vi "UI_Main.vi"() -> ()   [LabVIEW 2014]
panel:
  out "Resultant Vector":T1
  out "SpeedCap":dbl(slide) scale=0.18..1.0
  out "Pod Data Out":T2(array[cluster])
  in  "Speed Constraints":T3
  out "FZ":dbl(slide) scale=-1.0..1.0
  out "FXY":cluster{"X":dbl, "Y":dbl}[](graph)
  out "Swerve":picture
  in  "Pod Coordinates":cluster{"X":dbl, "Y":dbl}[](array[cluster])=[{"X"=2.0, "Y"=2.0}, {"X"=2.0, "Y"=-2.0}, {"X"=-2.0, "Y"=2.0}, {"X"=-2.0, "Y"=-2.0}]
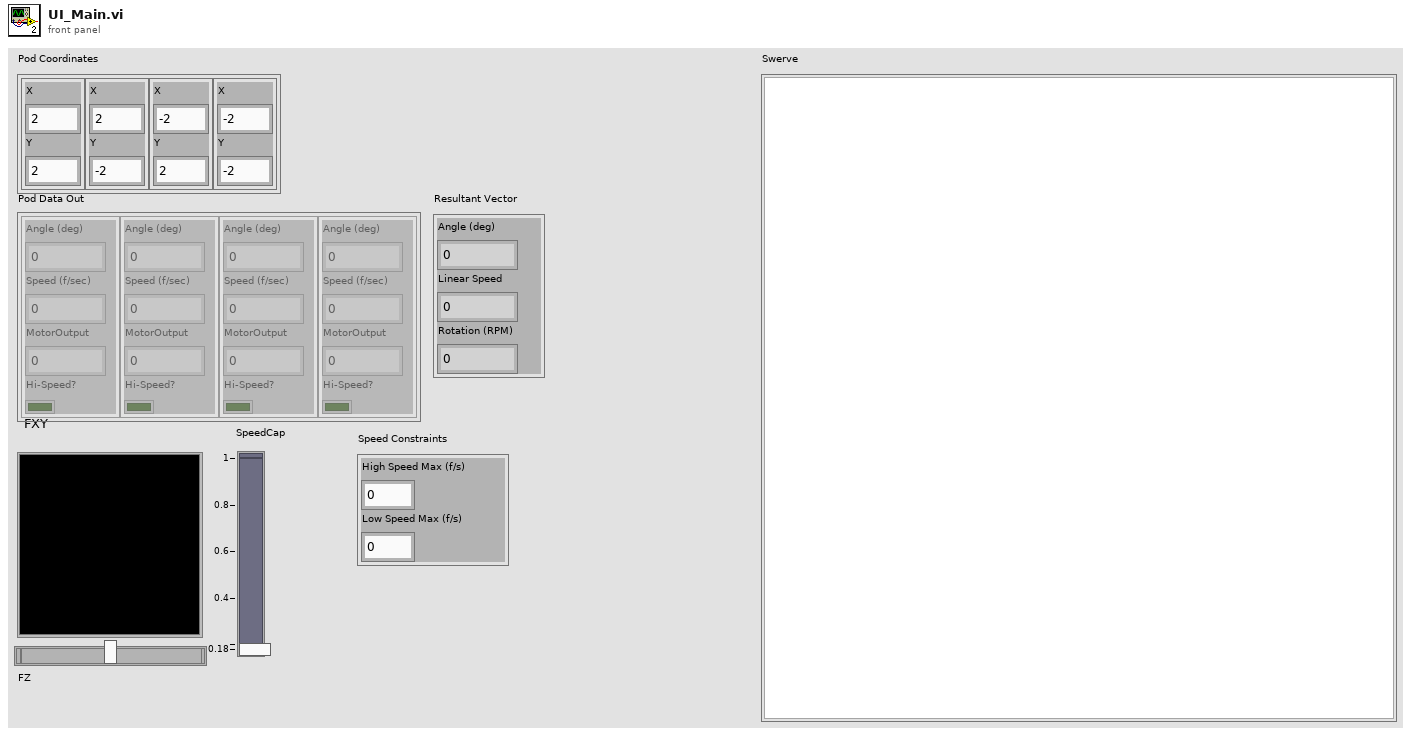
[diagram p1: front panel]
types:
  T1 = cluster{"Angle (deg)":dbl, "Linear Speed":dbl, "Rotation (RPM)":dbl}
  T2 = cluster{"Angle (deg)":dbl, "Speed (f/sec)":dbl, "MotorOutput":dbl, "Hi-Speed?":bool}[]
  T3 = cluster{"High Speed Max (f/s)":dbl, "Low Speed Max (f/s)":dbl}
  T4 = cluster{"Coords":cluster{"X":dbl, "Y":dbl}, "Vector":cluster{"X":dbl, "Y":dbl}, "Hi-Speed?":bool}[]
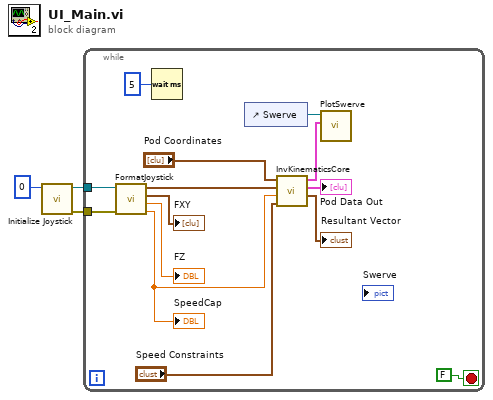
[diagram p0: block diagram]
diagram:
  n1 = call <vilib>:"Initialize Joystick.vi"("device index"=0) -> ("error out"=w1:errorcluster, "device ID"=w2:refnum<k1>)  [unwired: 9 in]
  n2 = while {
    tunnel: w2 -> [w14]
    tunnel: w1 -> [w13]
    stop <- FALSE stop-if-true
    n3 = call "FormatJoystick.vi"("error in (no error)"=w13, "Refnum in"=w14) -> ("Speed Cap"=w5:dbl, "FZ"=→"FZ":dbl, "FXY"=→"FXY":cluster{"X":dbl, "Y":dbl}[], "Axes"=w11:cluster{"X":dbl, "Y":dbl, "Z":dbl})  [unwired: 6 in]
    "SpeedCap" <- w5
    n4 = Wait (ms)(milliseconds to wait=u32 5) -> ()  [unwired: 1 out]
    n5 = control-ref of="Swerve"() -> (w17:refnum<vi>)
    n6 = call "InvKinematicsCore.vi"("Speed Constraints"="Speed Constraints", "Speed Cap"=w5, "Joystick Data"=w11, "Pod Coordinates"="Pod Coordinates") -> ("Resultant Vector"=→"Resultant Vector":T1, "Pod User Data Out"=→"Pod Data Out":T2, "Pod Plot Data Out"=w10:T4)  [unwired: 5 in]
    n7 = call "PlotSwerve.vi"("Pod Plot Data In"=w10, "Picture refrence"=w17) -> ()  [unwired: 10 in]
  }
